vi "习4.4.vi"() -> ()   [LabVIEW 2017]
panel:
  in  "数值":dbl
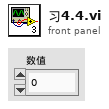
[diagram p1: front panel]
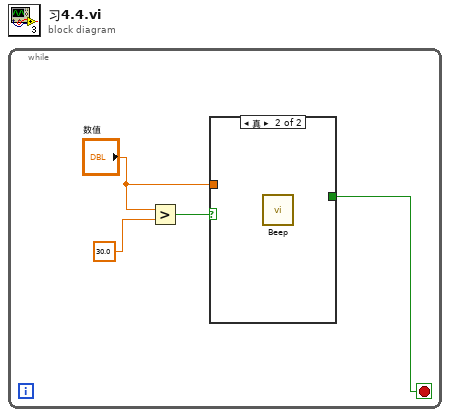
[diagram p0: block diagram]
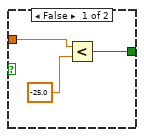
[diagram p2: hidden frame]
diagram:
  n1 = while {
    stop <- w1 stop-if-true
    n2 = Greater?(x="数值", y=30.0) -> (0:w3:bool)
    n3 = case shown="真" w3 {
      tunnel: "数值" -> [w6 _]
      tunnel: [w5 _] -> w1
      frame False {
        n4 = Less?(x=w6, y=-25.0) -> (x < y?=w5:bool)
      }
      frame True {
        n5 = call <vilib>:"Beep.vi"() -> ()  [unwired: 12 in]
      }
    }
  }
